vi "Initialize.vi"(8 "error in (no error)":errorcluster, 9 "Acquisition Rate":u16(ring)=100 items=["10"=10, "15"=15, "20"=20, "25"=25, "30"=30, "40"=40, "45"=45, "50"=50, "60"=60, "75"=75, "80"=80, "90"=90, "100"=100, "120"=120, "125"=125, "150"=150, "180"=180, "200"=200, "225"=225, "240"=240, "250"=250, "300"=300, "360"=360, "400"=400, "450"=450, "500"=500, "600"=600, "800"=800, "900"=900, "1000"=1000, "1200"=1200, "1500"=1500, "1800"=1800, "2000"=2000], 10 "ID Query (True)":bool=TRUE) -> (0 "error out":errorcluster, 1 "Device Count":i32)   [LabVIEW 2015, in "G 5.lvlib"]
uses:
  G 5.lvlib
  <vilib>/Platform/TimedLoop/XDataNode/timing_clust.ctl
  <vilib>/Platform/TimedLoop/XDataNode/nitl_modes.ctl
  <vilib>/Platform/TimedLoop/XDataNode/wakeup.ctl
  <vilib>/Platform/TimedLoop/XDataNode/XDataNode.xnode
  <vilib>/Platform/TimedLoop/XDataNode/XDNodeRunTimeDep.lvlib
  AMTIUSBDevice.dll
panel:
  in  "stop":bool
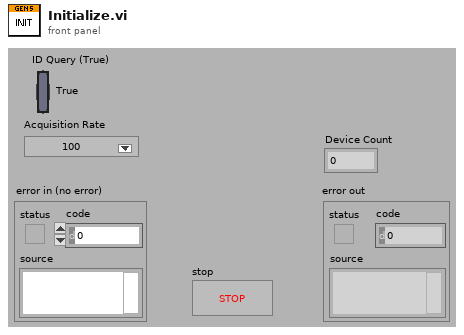
[diagram p1: front panel]
types:
  T1 = typedef "XDNodeRunTimeDep.lvlib/timing_clust.ctl" = cluster{"Expected End [f-1]":u64, "Actual End [f-1]":u64, "Finished Late? [f-1]":bool, "Expected End [i-1]":u64, "Actual End [i-1]":u64, "Finished Late? [i-1]":bool, "Expected Start [i]":u64, "Actual Start [i]":u64, "Expected Start [f]":u64, "Actual Start [f]":u64, "Source Name":string, "Structure Name":string, "Period":i64, "Deadline":i64, "Offset":i64, "Start":i64, "Priority":i32, "Timeout":i32, "Mode":T2, "Wakeup Reason":T3, "Error":errorcluster, "Source Type":string, "Secondary Source Type":string, "Global End Time":u64, "Global Start Time":u64, "Frame Duration":u64, "Iteration Duration":u64, "Assigned CPU":i32, "I/O Scan Engine Mode":u32}
  T2 = typedef "XDNodeRunTimeDep.lvlib/nitl_modes.ctl" = enum32{"No Change", "Process missed periods, maintain original phase", "Discard missed periods, maintain original phase", "Process missed periods, ignore original phase", "Discard missed periods, ignore original phase"}
  T3 = typedef "XDNodeRunTimeDep.lvlib/wakeup.ctl" = enum32{"Normal", "Aborted", "Asynchronous wakeup", "Timing source error", "Timed loop error", "Timeout"}
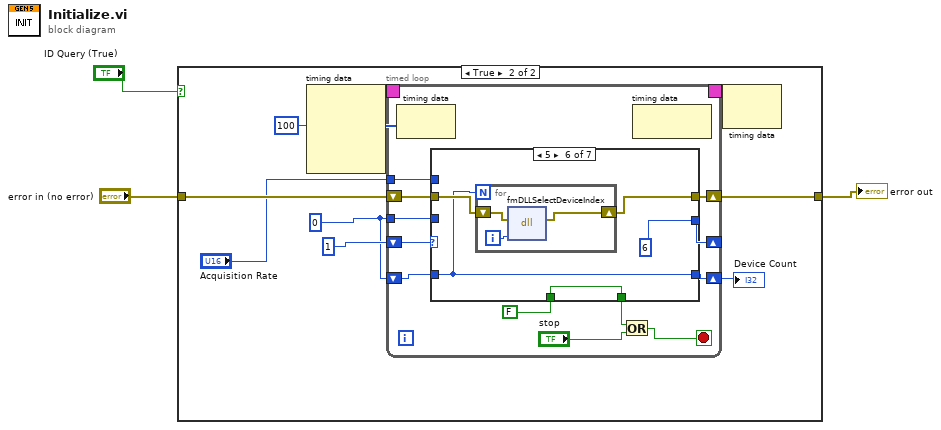
[diagram p0: block diagram]
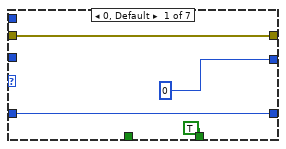
[diagram p3: hidden frame]
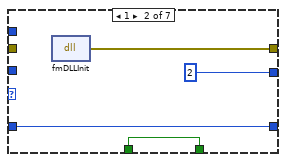
[diagram p4: hidden frame]
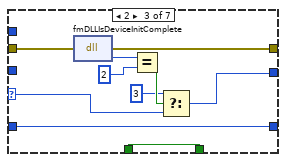
[diagram p5: hidden frame]
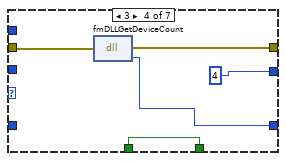
[diagram p6: hidden frame]
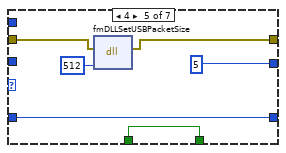
[diagram p7: hidden frame]
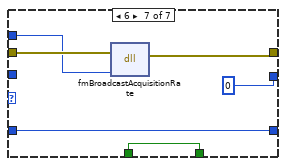
[diagram p8: hidden frame]
diagram:
  n1 = case shown="True" "ID Query (True)" {
    tunnel: [w4 w8] -> w1
    tunnel: "error in (no error)" -> [w4 w7]
    frame False {
    }
    frame True {
      w9 = 0
      n2 = node-c288(i64 100 ("Period")) -> (w13:T1)  [unwired: 3 in]
      n3 = timed-loop {
        shift-right: [w25] -> w8
        shift-left: w7 -> [w22]
        shift-right: [w23] -> _
        shift-left: 1 -> [w24]
        timing: w13 -> [_]
        timing-out: [_] -> w12
        tunnel: w9 -> [w21]
        shift-right: [w16] -> w6
        shift-left: w9 -> [w15]
        tunnel: "Acquisition Rate" -> [w14]
        stop <- w19 stop-if-true
        n4 = node-c288() -> ()  [unwired: 1 in, 1 out]
        n5 = case shown="5" w24 {
          selector: w24 -> [_ _ w40 _ _ _ _]
          tunnel: [w29 w35 w42 w49 w54 w58 w68] -> w25
          tunnel: [0 ("Numeric") 2 w38 4 5 6 0 ("Numeric")] -> w23
          tunnel: w22 -> [w29 _ w43 w50 w55 w59 w70]
          tunnel: w21 -> [_ _ _ _ _ _ _]
          tunnel: [TRUE w33 w37 w47 w52 w60 w65] -> w18
          tunnel: FALSE -> [_ w33 w37 w47 w52 w60 w65]
          tunnel: [w28 w32 w36 w46 w51 w57 w66] -> w16
          tunnel: w15 -> [w28 w32 w36 _ w51 w57 w66]
          tunnel: w14 -> [_ _ _ _ _ _ w69]
          frame 0, Default {
          }
          frame 1 {
            n6 = dll-call lib="AMTIUSBDevice.dll" fn="fmDLLInit"() -> (error out=w35:errorcluster)  [unwired: 4 in, 1 out]
          }
          frame 2 {
            n7 = dll-call lib="AMTIUSBDevice.dll" fn="fmDLLIsDeviceInitComplete"(error in=w43) -> (error out=w42:errorcluster, "InitComplete"=w44:i64)  [unwired: 2 in, 1 out]
            n8 = Equal?(x=w44, y=i64 2) -> (x = y?=w41:bool)
            n9 = Select(t=3, s=w41, f=w40) -> (s? t:f=w38:i32)
          }
          frame 3 {
            n10 = dll-call lib="AMTIUSBDevice.dll" fn="fmDLLGetDeviceCount"(error in=w50) -> (error out=w49:errorcluster, "DeviceCount"=w46:i32)  [unwired: 2 in, 1 out]
          }
          frame 4 {
            n11 = dll-call lib="AMTIUSBDevice.dll" fn="fmDLLSetUSBPacketSize" label="PacketSize"(error in=w55, "PacketSize"=512) -> (error out=w54:errorcluster)  [unwired: 4 in, 1 out]
          }
          frame 5 {
            n12 = for {
              N: w57 -> [_]
              shift-right: [w63] -> w58
              shift-left: w59 -> [w64]
              i -> [w62]
              n13 = dll-call lib="AMTIUSBDevice.dll" fn="fmDLLSelectDeviceIndex" label="SelectDeviceIndex"(error in=w64, "DeviceIndex"=w62) -> (error out=w63:errorcluster)  [unwired: 4 in, 1 out]
            }
          }
          frame 6 {
            n14 = dll-call lib="AMTIUSBDevice.dll" fn="fmBroadcastAcquisitionRate"(error in=w70, "ACQ Rate"=w69) -> (error out=w68:errorcluster)  [unwired: 4 in, 1 out]
          }
        }
        n15 = Or(x=w18, y="stop") -> (x .or. y?=w19:bool)
        n16 = node-c288() -> ()  [unwired: 1 in, 1 out]
      }
      "Device Count" <- w6
      n17 = node-c288(w12) -> ()  [unwired: 1 out]
    }
  }
  "error out" <- w1
